vi "SMSMagnet.destructor.vi"(0 "i ref in":refnum<vi>, 5 "error in (no error)":errorcluster) -> (19 "error out":errorcluster)   [LabVIEW 2014, in "SMSMagnet.lvlib"]
doc: "This is the destructor of a class.\n\nLicense Agreement for this software:\n\nCopyright (C)\nGesellschaft für Schwerionenforschung, GSI\nPlanckstr. 1\n64291 Darmstadt\nGermany\n\nContact: D.Beck@gsi.de \n\nThis program is free software; you can redistribute it and/or modify it under the terms of the \nGNU General Public License as published by the Free Software Foundation; either version 2 of \nthe license, or (at your option) any later version.\n\nThis program is distributed in the hope that it will be useful, but WITHOUT ANY WARRANTY; \nwithout even the implied warranty of MERCHANTABILITY or FITNESS FOR A PARTICULAR PURPOSE. See the GNU General License for more details (http://www.gnu.org).\n\nGesellschaft für Schwerionenforschung, GSI\nPlanckstr. 1, 64291 Darmstadt, Germany\nFor all questions and ideas contact: M.Richter@gsi.de, H.Brand@gsi.de or D.Beck@gsi.de.\nLast update: 16-JUN-2004"
uses:
  SMSMagnet.lvlib
  CS_Core/CSApplicationBaseClasses/DeviceBase/DeviceBase.lvlib
  CSlibraries-extern/DimLVEvent/LVDimInterface/LVDimInterface.lvlib
  instr.lib/SMSMagnetDriver/SMSMagnetDriver.lvlib
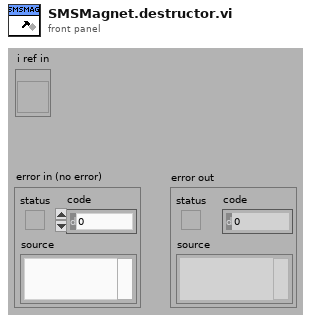
[diagram p1: front panel]
types:
  T1 = typedef "SMSMagnet.lvlib/SMSMagnet.i attribute.ctl" = cluster{"ActValueID":i32, "NomValueID":i32, "VISA resource name":refnum<visa-resource-name>, "ActValue":dbl, "VISAsem":T2}
  T2 = typedef "Semaphore RefNum" = refnum<k1>
  T3 = enum16{"SetAttribute", "GetAttribute", "CreateAttribute", "DestroyAttribute", "DestroyAllAtributes"}
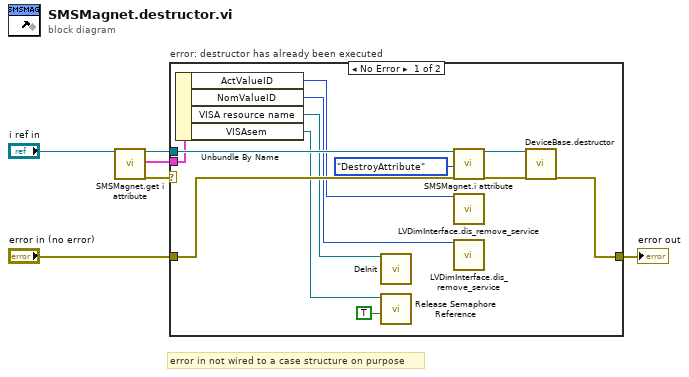
[diagram p0: block diagram]
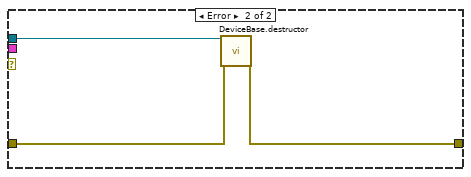
[diagram p2: hidden frame]
diagram:
  # "error in not wired to a case structure on purpose"
  n1 = call "SMSMagnet.get i attribute.vi"("i ref in"="i ref in") -> ("i ref out"=w2:refnum<vi>, "i attribute"=w1:T1, "error out"=w3:errorcluster)  [unwired: 16 in]
  n2 = case "error: destructor has already been executed" shown="No Error" w3 {
    tunnel: [w15 w19] -> w6
    tunnel: "error in (no error)" -> [w14 w20]
    tunnel: w2 -> [w13 w21]
    tunnel: w1 -> [w12 _]
    frame No Error {
      n3 = Unbundle By Name(w12) -> ("ActValueID"=w11:i32, "NomValueID"=w10:i32, "VISA resource name"=w9:refnum<visa-resource-name>, "VISAsem"=w8:T2)
      n4 = call "DeInit.vi"("VISA resource name"=w9) -> ()  [unwired: 18 in, 1 out]
      n5 = call <vilib>:"Release Semaphore Reference.vi"("force destroy? (F)"=TRUE, "semaphore"=w8) -> ()  [unwired: 8 in, 2 out]
      n6 = call "SMSMagnet.i attribute.vi"("VI Refnum"=w13, "Action"=T3."DestroyAttribute", "error in (no error)"=w14) -> ("VI Refnum out"=w17:refnum<vi>, "error out"=w16:errorcluster)  [unwired: 14 in, 1 out]
      n7 = call "LVDimInterface.dis_remove_service.vi"("my_serviceID"=w11) -> ()  [unwired: 18 in, 1 out]
      n8 = call "LVDimInterface.dis_remove_service.vi"("my_serviceID"=w10) -> ()  [unwired: 18 in, 1 out]
      n9 = call "DeviceBase.destructor.vi"("i ref in"=w17, "error in (no error)"=w16) -> ("error out"=w15:errorcluster)  [unwired: 17 in]
    }
    frame Error {
      n10 = call "DeviceBase.destructor.vi"("i ref in"=w21, "error in (no error)"=w20) -> ("error out"=w19:errorcluster)  [unwired: 17 in]
    }
  }
  "error out" <- w6
